vi "Set Overpressure Strategy.vi"(8 "error in (no error)":errorcluster, 11 "ASIA Pump #":i32) -> (0 "error out":errorcluster, 2 "strategySet":bool, 3 "ASIA Pump #":i32)   [LabVIEW 2018, in "ASIA Pump.lvlib" / "ASIA Support VIs.lvlib"]
uses:
  ASIA Support VIs.lvlib
  Third Party Drivers/4600031 - Version 1.2-Asia Pump Drivers/AsiaPumpInterface.dll
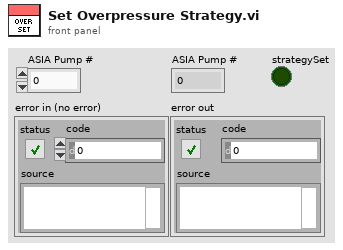
[diagram p1: front panel]
types:
  T1 = cluster{"Busy":bool, "PumpCnt":dbl, "RemoteEntered":bool, "OverpressureSet":bool}[]
  T2 = cluster{"Busy":bool, "PumpCnt":dbl, "RemoteEntered":bool, "OverpressureSet":bool}
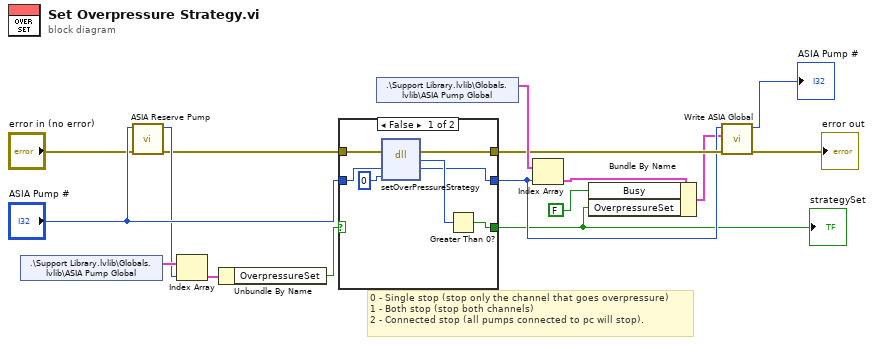
[diagram p0: block diagram]
diagram:
  # "0 - Single stop (stop only the channel that goes overpressure)\n1 - Both stop (stop both channels)\n2 - Connected stop (all pumps connected to pc will stop)."
  n1 = shared-variable ".\\Support Library.lvlib\\Globals.lvlib\\ASIA Pump Global"() -> (w16:T1)  [unwired: 1 in, 1 out]
  n2 = call "ASIA Reserve Pump.vi"("error in (no error)"="error in (no error)", "ASIA Pump #"="ASIA Pump #") -> ("error out"=w10:errorcluster, "ASIA Pump #"=w12:i32)  [unwired: 8 in]
  n3 = Index Array(array=w16, index=w12) -> (element=w15:T2)
  n4 = Unbundle By Name(w15) -> ("OverpressureSet"=w14:bool)
  n5 = case shown="False" w14 {
    selector: w14 -> [_ w26]
    tunnel: w10 -> [w22 w24]
    tunnel: "ASIA Pump #" -> [w21 w25]
    tunnel: [w19 w26] -> w4
    tunnel: [w18 w25] -> w6
    tunnel: [w17 w24] -> w7
    frame False {
      n6 = dll-call lib="C:/Users/FAST Lab/Documents/LabVIEW Data/Projects/Pfizer Timed Seq/Third Party Drivers/4600031 - Version 1.2-Asia Pump Drivers/AsiaPumpInterface.dll" fn="setOverPressureStrategy"(error in=w22, "pumpNum"=w21, "strategy"=u8 0) -> (error out=w17:errorcluster, "Bool"=w20:u8, "pumpNum"=w18:u32)  [unwired: 3 in, 1 out]
      n7 = Greater Than 0?(x=w20) -> (x > 0?=w19:bool)
    }
    frame True {
    }
  }
  "strategySet" <- w4
  n8 = shared-variable ".\\Support Library.lvlib\\Globals.lvlib\\ASIA Pump Global"() -> (w8:T1)  [unwired: 1 in, 1 out]
  n9 = Index Array(array=w8, index=w6) -> (element=w9:T2)
  n10 = Bundle By Name(cluster=w9, "Busy"=FALSE, "OverpressureSet"=w4) -> (w1:T2)
  n11 = call "Write ASIA Global.vi"("error in (no error)"=w7, "ASIA Global"=w1, "Pump Number"=w6) -> ("error out"=→"error out":errorcluster, "Pump Number"=→"ASIA Pump #":i32)  [unwired: 7 in]
